vi "Real Inverse Matrix (LU).vi"(0 "A":T1) -> (1 "Inverse Matrix":T1, 2 "error":i32)   [LabVIEW 2017, in "NI_AALBase.lvlib"]
uses:
  <vilib>/Analysis/NI_AALBase.lvlib
  <vilib>/Analysis/Matrix/Datatypes/RealMatrix.ctl
  <resource>/lvanlys.dll
  <vilib>/Analysis/Matrix/NI_Matrix.lvlib
panel:
  # "Real Inverse Matrix (LU)"
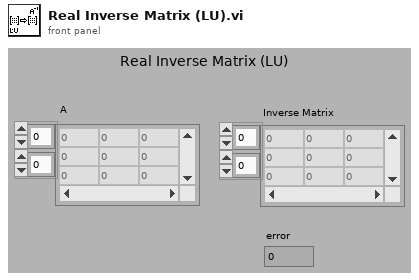
[diagram p1: front panel]
types:
  T1 = typedef "NI_Matrix.lvlib/RealMatrix.ctl" = dbl[][]
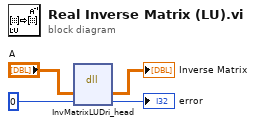
[diagram p0: block diagram]
diagram:
  n1 = dll-call lib="e:/builds/penguin/labview/branches/2017/dev/dist/resource/lvanlys.*" fn="InvMatrixLUDri_head"("A"="A", "error"=0) -> ("A"=→"Inverse Matrix":T1, "error"=→"error":i32)  [unwired: 4 in, 2 out]
